vi "Depth Array To Image.vi"(4 "Image Dest.":T1, 5 "Depth Array":u16[][](array[numeric])) -> (1 "Image out":T1)   [LabVIEW 2018]
uses:
  <vilib>/vision/Image Controls.llb/IMAQ Image.ctl
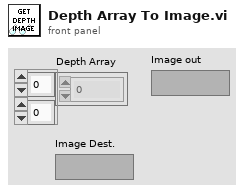
[diagram p1: front panel]
types:
  T1 = typedef "IMAQ Image.ctl" = refnum<image>
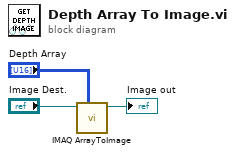
[diagram p0: block diagram]
diagram:
  n1 = call "IMAQ ArrayToImage"("Image Pixels (U16)"="Depth Array", "Image"="Image Dest.") -> ("Image Out"=→"Image out":T1)  [unwired: 8 in, 1 out]
